vi "Ramp Navigation Loop.vi"() -> ()   [LabVIEW 2009]
uses:
  Remote Control/Motor Command.ctl
  <vilib>/Platform/TimedLoop/XDataNode/XDataNode.xnode
  <vilib>/Platform/TimedLoop/XDataNode/loadlvalarms.vi
  <vilib>/Platform/TimedLoop/XDataNode/timing_clust.ctl
  <vilib>/Platform/TimedLoop/XDataNode/nitl_modes.ctl
  <vilib>/Platform/TimedLoop/XDataNode/wakeup.ctl
  <vilib>/Analysis/3filter.llb/Filter Passband Type.ctl
  cRIO/Functional Global Variables/Actions for FG's.ctl
  <vilib>/Analysis/3filter.llb/Butterworth Filter (DBL).vi
  <vilib>/Platform/TimedLoop/XDataNode/XDNodeRunTimeDep.lvlib
  <vilib>/Analysis/NI_AALBase.lvlib
panel:
  in  "On Ramp in":bool=TRUE
  in  "Roll offset":dbl=0.9
  in  "Pitch offset":dbl=2.6
  out "Slide":i16(slide) scale=-10.0..10.0
  out "On Ramp?":bool
  out "Waveform Chart 2":cluster{"mean":dbl, "mean":dbl}(graph)
  out "Waveform Chart":T1(graph)
  out "Roll Buffer out":dbl
  out "Pitch Buffer out":dbl
  out "Absolute tilt of surface":dbl
  out "Motor Commands":T2
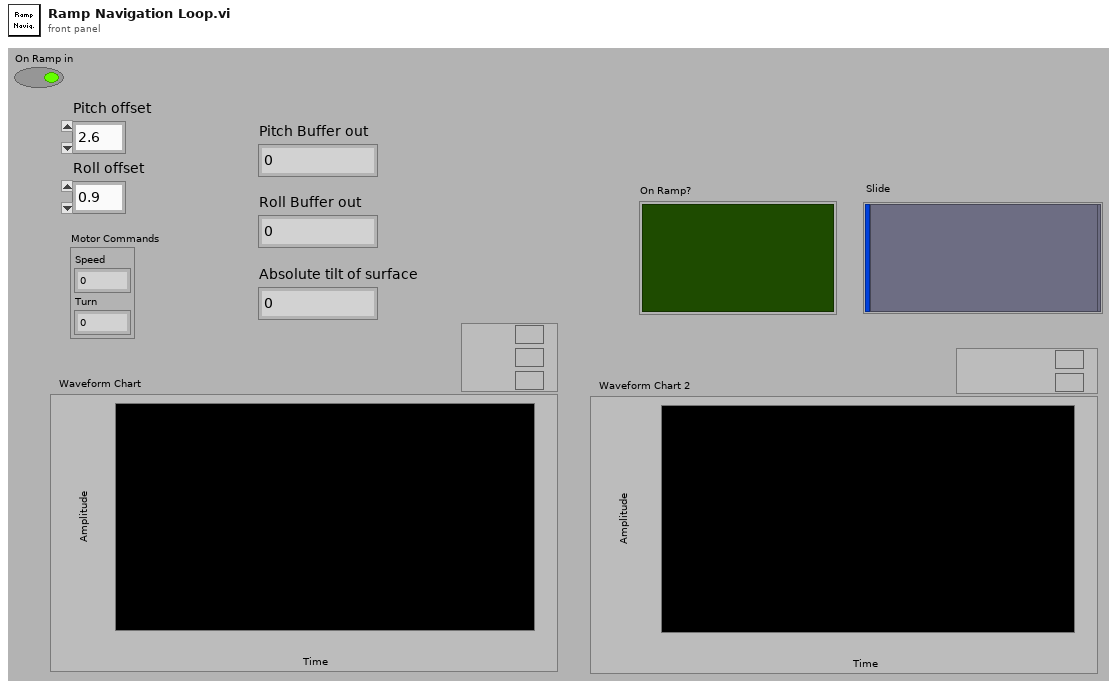
[diagram p1: front panel]
types:
  T1 = cluster{dbl, "Pitch Buffer out":dbl, "Roll Buffer out":dbl}
  T2 = typedef "Motor Command.ctl" = cluster{"Speed":i16, "Turn":i16}
  T3 = typedef "XDNodeRunTimeDep.lvlib/timing_clust.ctl" = cluster{"Expected End [f-1]":u64, "Actual End [f-1]":u64, "Finished Late? [f-1]":bool, "Expected End [i-1]":u64, "Actual End [i-1]":u64, "Finished Late? [i-1]":bool, "Expected Start [i]":u64, "Actual Start [i]":u64, "Expected Start [f]":u64, "Actual Start [f]":u64, "Source Name":string, "Structure Name":string, "Period":i64, "Deadline":i64, "Offset":i64, "Start":i64, "Priority":i32, "Timeout":i32, "Mode":T4, "Wakeup Reason":T5, "Error":errorcluster, "Source Type":string, "Secondary Source Type":string, "Global End Time":u64, "Global Start Time":u64, "Frame Duration":u64, "Iteration Duration":u64, "Assigned CPU":i32, "I/O Scan Engine Mode":u32}
  T4 = typedef "XDNodeRunTimeDep.lvlib/nitl_modes.ctl" = enum32{"No Change", "Process missed periods, maintain original phase", "Discard missed periods, maintain original phase", "Process missed periods, ignore original phase", "Discard missed periods, ignore original phase"}
  T5 = typedef "XDNodeRunTimeDep.lvlib/wakeup.ctl" = enum32{"Normal", "Aborted", "Asynchronous wakeup", "Timing source error", "Timed loop error", "Timeout"}
  T6 = typedef "NI_AALBase.lvlib/Filter Passband Type.ctl" = enum32{"Lowpass", "Highpass", "Bandpass", "Bandstop"}
  T7 = typedef "Actions for FG's.ctl" = enum16{"Read", "Write"}
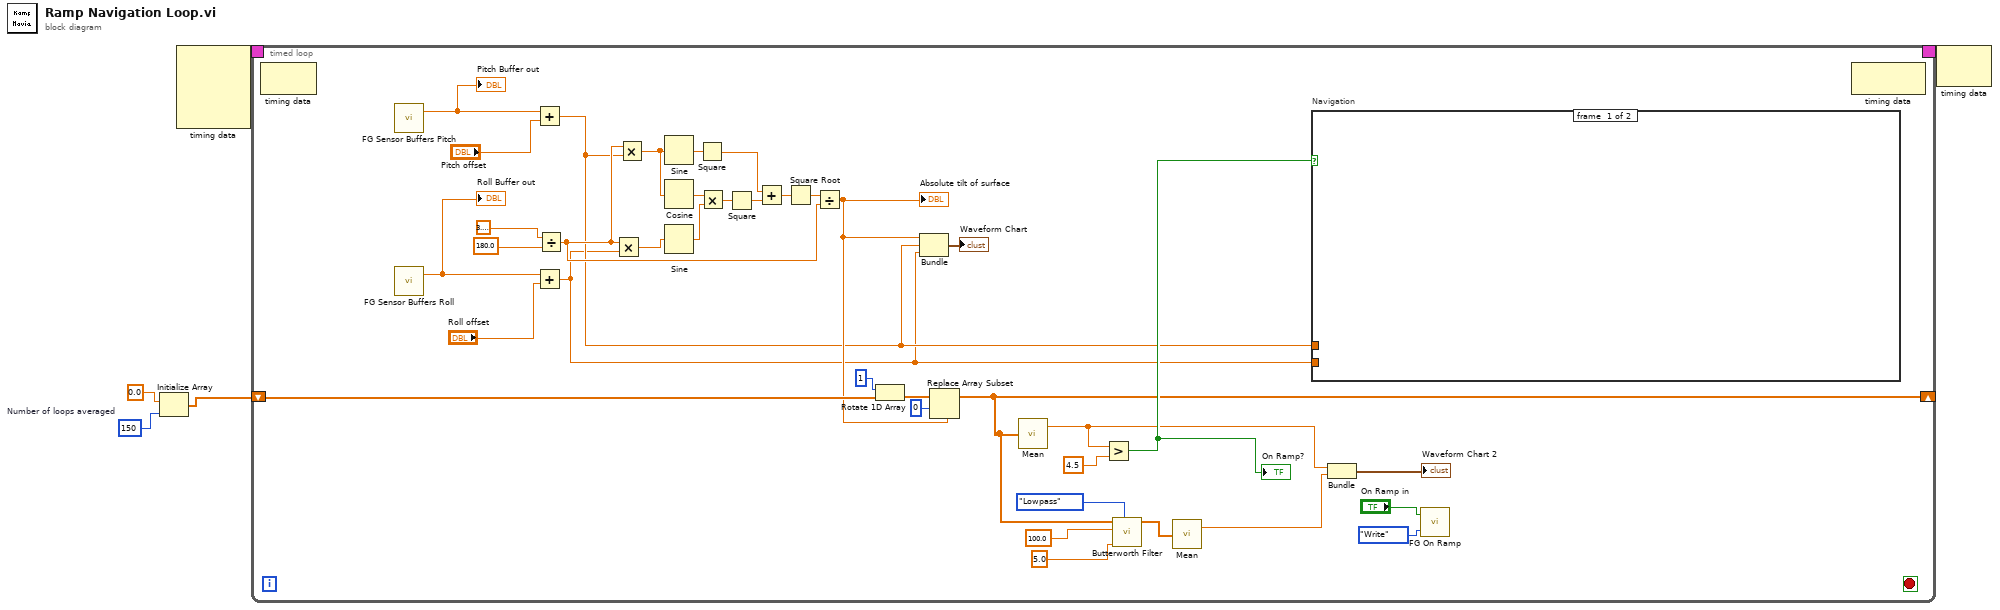
[diagram p0: block diagram]
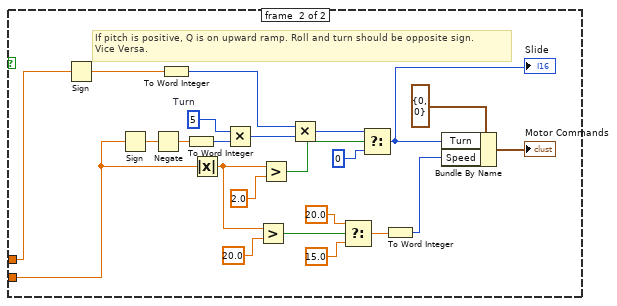
[diagram p2: hidden frame]
diagram:
  w2 = 150  # Number of loops averaged
  n1 = Initialize Array(0.0 ("element"), w2) -> (w1:dbl[])
  n2 = node-c288() -> (w5:T3)  [unwired: 4 in]
  n3 = timed-loop {
    timing: w5 -> [_]
    timing-out: [_] -> w4
    shift-right: [w14] -> _
    shift-left: w1 -> [w25]
    stop <- _ stop-if-true
    n4 = node-c288() -> ()  [unwired: 1 in, 1 out]
    n5 = call "FG Sensor Buffers Pitch.vi"() -> ("Pitch Buffer out"=w18:dbl)  [unwired: 3 in]
    "Pitch Buffer out" <- w18
    n6 = call "FG Sensor Buffers Roll.vi"() -> ("Roll Buffer out"=w26:dbl)  [unwired: 3 in]
    "Roll Buffer out" <- w26
    n7 = Add(x=w18, y="Pitch offset") -> (x+y=w16:dbl)
    n8 = Add(x=w26, y="Roll offset") -> (x+y=w15:dbl)
    n9 = Divide(x=3.141592653589793, y=180.0) -> (x/y=w30:dbl)
    n10 = Multiply(x=w30, y=w15) -> (x*y=w32:dbl)
    n11 = Multiply(x=w30, y=w16) -> (x*y=w33:dbl)
    n12 = Sine(x=w33) -> (sin(x)=w39:dbl)
    n13 = Cosine(x=w33) -> (cos(x)=w41:dbl)
    n14 = Sine(x=w32) -> (sin(x)=w42:dbl)
    n15 = Square(x=w39) -> (x^2=w38:dbl)
    n16 = Multiply(x=w41, y=w42) -> (x*y=w40:dbl)
    n17 = Square(x=w40) -> (x^2=w37:dbl)
    n18 = Add(x=w38, y=w37) -> (x+y=w36:dbl)
    n19 = Square Root(x=w36) -> (sqrt(x)=w31:dbl)
    n20 = Divide(x=w31, y=w30) -> (x/y=w21:dbl)
    "Absolute tilt of surface" <- w21
    n21 = Rotate 1D Array(1:w25, 2:1 ("n")) -> (0:w23:dbl[])
    n22 = Bundle(w21, w16, w15) -> (→"Waveform Chart":cluster{dbl, dbl, dbl})  [unwired: 1 in]
    n23 = Replace Array Subset(array=w23, new element=w21, index=0) -> (w14:dbl[])
    n24 = call <vilib>:"Mean.vi"("X"=w14) -> ("mean"=w9:dbl)  [unwired: 1 out]
    n25 = Greater?(x=w9, y=4.5) -> (0:w17:bool)
    "On Ramp?" <- w17
    n26 = call-poly <vilib>:"Butterworth Filter.vi"("filter type"=Filter_Passband_Type."Lowpass", "low cutoff freq: fl"=5.0 ("high cutoff freq: fh"), "sampling freq: fs"=100.0, "X"=w14) -> ("Filtered X"=w10:dbl[])  [unwired: 4 in, 1 out]
    n27 = call <vilib>:"Mean.vi"("X"=w10) -> ("mean"=w8:dbl)  [unwired: 1 out]
    n28 = case "Navigation" shown="True" w17 {
      tunnel: w15 -> [_ w50]
      tunnel: w16 -> [_ w48]
      frame #0 {
      }
      frame #1 {
        w49 = i16 5  # Turn
        # "If pitch is positive, Q is on upward ramp. Roll and turn should be opposite sign.\nVice Versa."
        n29 = Sign(1:w48) -> (0:w45:dbl)
        n30 = Sign(1:w50) -> (0:w63:dbl)
        n31 = Negate(x=w63) -> (-x=w62:dbl)
        n32 = To Word Integer(number=w45) -> (16bit integer=w44:i16)
        n33 = To Word Integer(number=w62) -> (16bit integer=w54:i16)
        n34 = Absolute Value(x=w50) -> (abs(x)=w56:dbl)
        n35 = Multiply(x=w49, y=w54) -> (x*y=w46:i16)
        n36 = Greater?(x=w56, y=20.0) -> (0:w60:bool)
        n37 = Greater?(x=w56, y=2.0) -> (0:w55:bool)
        n38 = Multiply(x=w44, y=w46) -> (x*y=w47:i16)
        n39 = Select(t=20.0, s=w60, f=15.0) -> (s? t:f=w52:dbl)
        n40 = Select(t=w47, s=w55, f=i16 0) -> (s? t:f=w43:i16)
        "Slide" <- w43
        n41 = To Word Integer(number=w52) -> (16bit integer=w51:i16)
        n42 = Bundle By Name(cluster=T2 {"Speed"=0, "Turn"=0} ("Motor Command"), "Turn"=w43, "Speed"=w51) -> (→"Motor Commands":T2)
      }
    }
    n43 = Bundle("mean"=w9, "mean"=w8) -> (→"Waveform Chart 2":cluster{"mean":dbl, "mean":dbl})  [unwired: 1 in]
    n44 = call "FG On Ramp.vi"("FG Action"=Actions_for_FG's."Write", "On Ramp in"="On Ramp in") -> ()  [unwired: 1 in, 1 out]
    n45 = node-c288() -> ()  [unwired: 1 in, 1 out]
  }
  n46 = node-c288(w4) -> ()  [unwired: 1 out]
